vi "generate_unique_stabilisation_filename.vi"(10 "cell label":string, 11 "Data Folder":path) -> (3 "Filename":path)   [LabVIEW 2016]
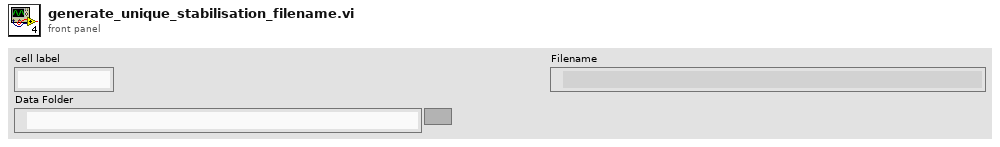
[diagram p1: front panel]
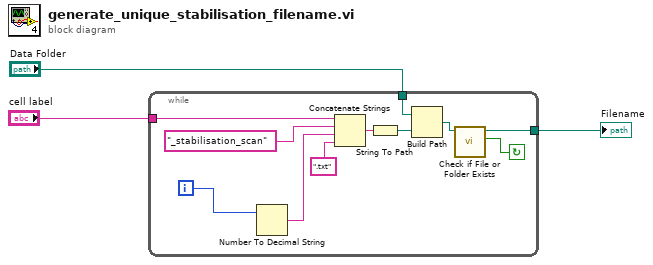
[diagram p0: block diagram]
diagram:
  n1 = while {
    tunnel: "cell label" -> [w14]
    tunnel: [w7] -> w1
    tunnel: "Data Folder" -> [w5]
    i -> [w12]
    stop <- w8 continue-if-true
    n2 = Number To Decimal String(number=w12) -> (decimal integer string=w11:string)  [unwired: 1 in]
    n3 = Concatenate Strings(w14, "_stabilisation_scan", w11, ".txt") -> (w9:string)
    n4 = String To Path(string=w9) -> (path=w6:path)
    n5 = Build Path(base path=w5, name or relative path=w6) -> (appended path=w4:path)
    n6 = call <vilib>:"Check if File or Folder Exists.vi"("path"=w4) -> ("file or folder exists?"=w8:bool, "dup path"=w7:path)  [unwired: 8 in, 1 out]
  }
  "Filename" <- w1
